vi "x_y(F.L).vi"(6 "Sensor 4":dbl, 7 "Array":dbl[](array[numeric]), 9 "Sensor 3":dbl, 10 "Sensor 2":dbl, 11 "Sensor 1":dbl) -> (1 "Sum (F.L)":dbl, 2 "y(F.L)":dbl, 3 "x(F.L)":dbl)   [LabVIEW 2019]
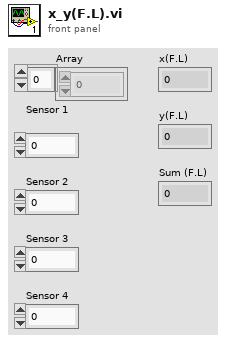
[diagram p1: front panel]
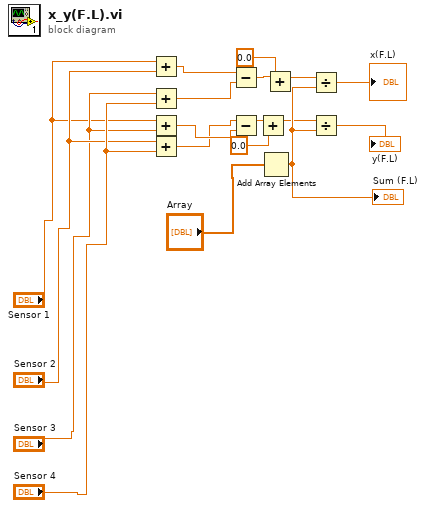
[diagram p0: block diagram]
diagram:
  n1 = Add(x="Sensor 1", y="Sensor 2") -> (x+y=w6:dbl)
  n2 = Add(x="Sensor 3", y="Sensor 4") -> (x+y=w5:dbl)
  n3 = Add(x="Sensor 1", y="Sensor 3") -> (x+y=w8:dbl)
  n4 = Add(x="Sensor 2", y="Sensor 4") -> (x+y=w7:dbl)
  n5 = Subtract(x=w6, y=w5) -> (x-y=w11:dbl)
  n6 = Subtract(x=w7, y=w8) -> (x-y=w12:dbl)
  n7 = Add(x=w12, y=0.0) -> (x+y=w2:dbl)
  n8 = Add Array Elements(numeric array="Array") -> (sum=w9:dbl)
  "Sum (F.L)" <- w9
  n9 = Add(x=w11, y=0.0) -> (x+y=w4:dbl)
  n10 = Divide(x=w4, y=w9) -> (x/y=→"x(F.L)":dbl)
  n11 = Divide(x=w2, y=w9) -> (x/y=→"y(F.L)":dbl)
